vi "Test parameters.vi"() -> ()   [LabVIEW 2015]
uses:
  RUS Parameters.ctl
panel:
  out "Update rate":i32
  in  "Samples per read":i32=1024
  out "Decimation":u64
  out "Frequencies":dbl[](array[numeric])
  in  "Parameters":T1={"Start frequency"=500000.0, "End frequency"=1500000.0, "Duration"=40.0, "Averaging"=0.0084, "Find peaks"=FALSE} {"Averaging" format="%#_8p"; "Duration" format="%#_6p"; "End frequency" format="%#_6p"; "Start frequency" format="%#_6p"}
  # "s"
  # "Hz"
  # "s"
  # "Hz"
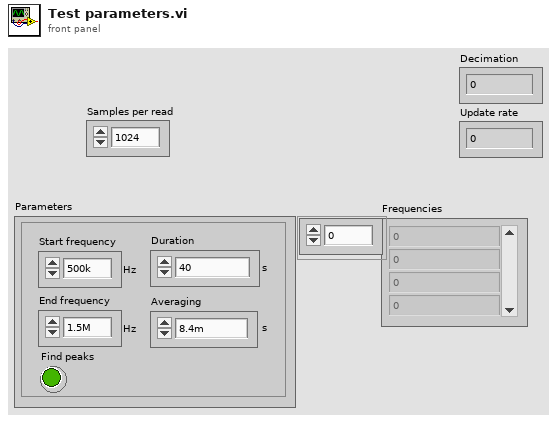
[diagram p1: front panel]
types:
  T1 = typedef "RUS Parameters.ctl" = cluster{"Start frequency":dbl, "End frequency":dbl, "Duration":dbl, "Averaging":dbl, "Find peaks":bool}
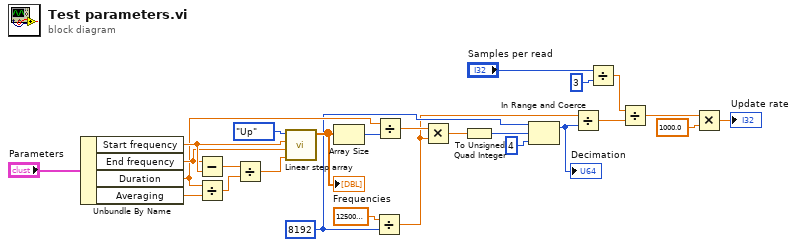
[diagram p0: block diagram]
diagram:
  w11 = u64 8192 ("x")
  n1 = Unbundle By Name("Parameters") -> ("Start frequency"=w23:dbl, "End frequency"=w22:dbl, "Duration"=w12:dbl, "Averaging"=w21:dbl)
  n2 = Subtract(x=w22, y=w23) -> (x-y=w24:dbl)
  n3 = Divide(x=w12, y=w21) -> (x/y=w25:dbl)
  n4 = Divide(x=w24, y=w25) -> (x/y=w26:dbl)
  n5 = call "Linear step array.vi"("Step"=w26, "End"=w22, "Start"=w23, "Mode"=enum16{"Up", "Up-down"}."Up") -> ("Steps"=w13:dbl[])  [unwired: 7 in]
  "Frequencies" <- w13
  n6 = Array Size(array=w13) -> (size(s)=w14:i32)
  n7 = Divide(x=125000000.0 ("y"), y=w11) -> (x/y=w3:dbl)
  n8 = Divide(x=w12, y=w14) -> (x/y=w18:dbl)
  n9 = Multiply(x=w18, y=w3) -> (x*y=w17:dbl)
  n10 = To Unsigned Quad Integer(1:w17) -> (0:w15:u64)
  n11 = In Range and Coerce(upper limit=w11, x=w15, lower limit=u64 4 ("Command payload")) -> (coerced(x)=w2:u64)  [unwired: 1 out]
  "Decimation" <- w2
  n12 = Divide(x=w3, y=w2) -> (x/y=w6:dbl)
  n13 = Divide(x="Samples per read", y=3) -> (x/y=w5:dbl)
  n14 = Divide(x=w5, y=w6) -> (x/y=w7:dbl)
  n15 = Multiply(x=w7, y=1000.0) -> (x*y=→"Update rate":dbl)
